vi "tsdiag_can_communication_control.vi"(8 "ATimeOutMs":i32, 9 "AControlType":u8, 10 "ADiagModuleIndex":i32, 11 "路径输入":path) -> (2 "返回类型":i32, 3 "路径输出":path)   [LabVIEW 2019]
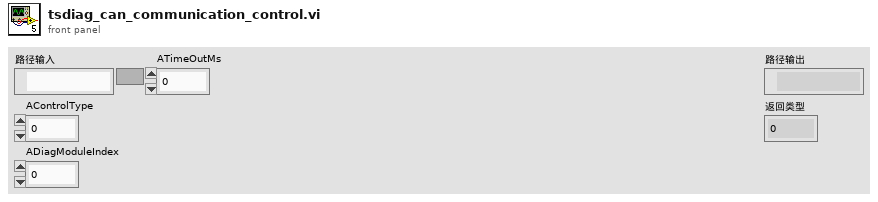
[diagram p1: front panel]
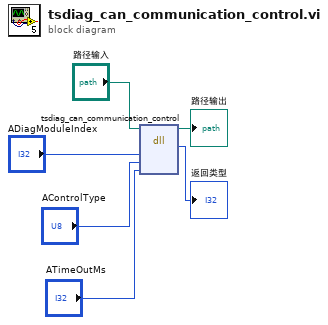
[diagram p0: block diagram]
diagram:
  n1 = dll-call lib="C:/Users/XYY/Desktop/LabView Demo/TSCAN_LB2018_V1.4_20220309/Config/TSMaster.dll" fn="tsdiag_can_communication_control"(path in="路径输入", "ADiagModuleIndex"="ADiagModuleIndex", "AControlType"="AControlType", "ATimeOutMs"="ATimeOutMs") -> (path out=→"路径输出":path, "返回类型"=→"返回类型":i32)  [unwired: 5 in, 1 out]
